vi "Duplicate Disabled Frame.vi"(8 "Error In":errorcluster, 11 "DisableStructure In":refnum<vi>) -> (0 "Error Out":errorcluster, 3 "DisableStructure Out":refnum<vi>)   [LabVIEW 2017, in "Eulogy.lvlib"]
uses:
  Eulogy.lvlib
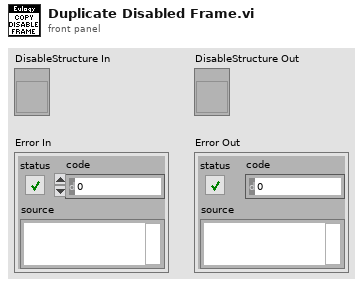
[diagram p1: front panel]
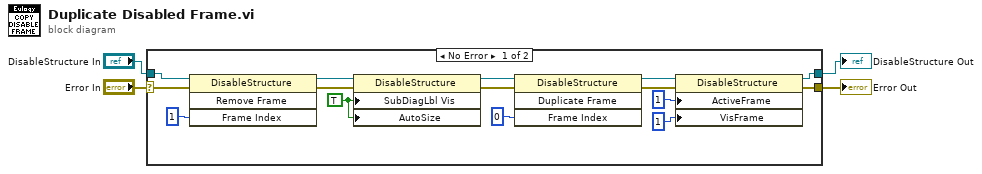
[diagram p0: block diagram]
diagram:
  n1 = case shown="No Error" "Error In" {
    selector: "Error In" -> [w5 w20]
    tunnel: [w16 w21] -> w4
    tunnel: [w11 w20] -> w3
    tunnel: "DisableStructure In" -> [w6 w21]
    frame No Error {
      w19 = TRUE ("Subdiagram Label Visible")
      n2 = invoke class="DisableStructure" method="Remove Frame"(reference=w6, error in=w5, "Frame Index"=u32 1) -> (reference out=w7:refnum<vi>, error out=w14:errorcluster)  [unwired: 1 in, 2 out]
      n3 = property class="DisableStructure"(reference=w7, error in=w14, "SubDiagLbl Vis"=w19, "AutoSize"=w19) -> (reference out=w13:refnum<vi>, error out=w15:errorcluster)
      n4 = invoke class="DisableStructure" method="Duplicate Frame"(reference=w13, error in=w15, "Frame Index"=u32 0) -> (reference out=w12:refnum<vi>, error out=w9:errorcluster)  [unwired: 1 in, 2 out]
      n5 = property class="DisableStructure"(reference=w12, error in=w9, "ActiveFrame"=i16 1 ("Active Frame"), "VisFrame"=u32 1 ("Visible Frame")) -> (reference out=w16:refnum<vi>, error out=w11:errorcluster)
    }
    frame Error {
    }
  }
  "DisableStructure Out" <- w4
  "Error Out" <- w3
